vi "题4.4.vi"() -> ()   [LabVIEW 2017]
uses:
  <vilib>/Analysis/2dsp.llb/Real FFT.vi
  <vilib>/Analysis/NI_AALPro.lvlib
  <vilib>/measure/NI_MABase.lvlib
panel:
  out "时域信号":dbl[](graph)
  out "频域信号":dbl[](graph)
  in  "frequency 3":dbl=10.0 caption="频率" format="%0.2p"
  in  "amplitude 3":dbl=1.0 caption="幅值" format="%0.2p"
  in  "amplitude 2":dbl=1.0 caption="幅值" format="%0.2p"
  in  "frequency 2":dbl=10.0 caption="频率" format="%0.2p"
  in  "amplitude":dbl=1.0 caption="幅值" format="%0.2p"
  in  "frequency":dbl=10.0 caption="频率" format="%0.2p"
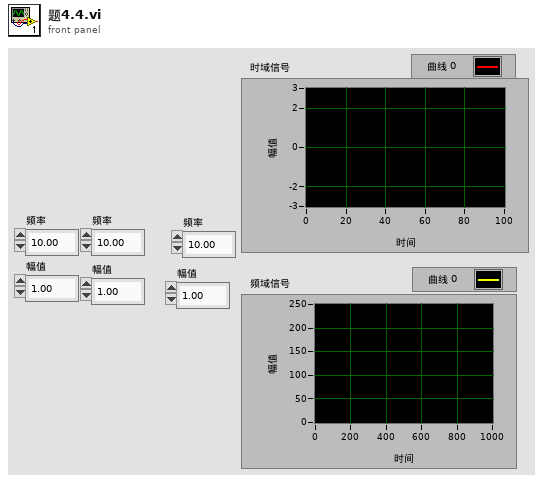
[diagram p1: front panel]
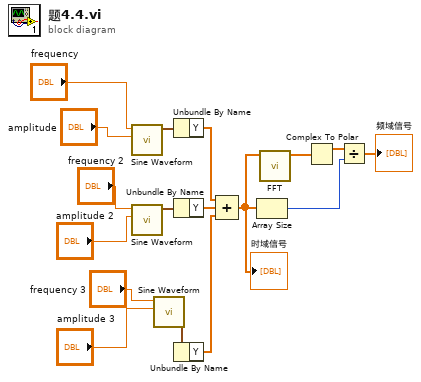
[diagram p0: block diagram]
diagram:
  n1 = call <vilib>:"Sine Waveform.vi"("amplitude"="amplitude", "frequency"="frequency") -> ("signal out"=w10:waveform(dbl))  [unwired: 8 in, 1 out]
  n2 = call <vilib>:"Sine Waveform.vi"("amplitude"="amplitude 2", "frequency"="frequency 2") -> ("signal out"=w9:waveform(dbl))  [unwired: 8 in, 1 out]
  n3 = call <vilib>:"Sine Waveform.vi"("amplitude"="amplitude 3", "frequency"="frequency 3") -> ("signal out"=w8:waveform(dbl))  [unwired: 8 in, 1 out]
  n4 = Unbundle By Name(w10) -> ("Y"=w7:dbl[])
  n5 = Unbundle By Name(w9) -> ("Y"=w6:dbl[])
  n6 = Unbundle By Name(w8) -> ("Y"=w5:dbl[])
  n7 = Compound Arithmetic op=ADD(w7, w6, w5) -> (w1:dbl[])
  "时域信号" <- w1
  n8 = Array Size(array=w1) -> (size(s)=w3:i32)
  n9 = call-poly <vilib>:"FFT.vi"("X"=w1) -> ("FFT {X}"=w11:cdb[])  [unwired: 9 in, 1 out]
  n10 = Complex To Polar(r * e^(i*theta)=w11) -> (r=w4:dbl[])  [unwired: 1 out]
  n11 = Divide(x=w4, y=w3) -> (x/y=→"频域信号":dbl[])
